vi "RandomFlag vs UUID Flag.vi"() -> ()   [LabVIEW 2020]
uses:
  <userlib>/_NEVSTOP/Communicable State Machine(CSM)/Communicable State Machine.lvlib
panel:
  out "UUID Flag":string
  out "Random Flag":u64
  out "unit (ms) 2":dbl[](graph)
  out "inside 2":i32
  out "outside 2":i32
  out "inside":i32
  out "outside":i32
  out "unit (ms)":dbl[][](graph)
  # "RandomFlag vs UUID Flag.vi"
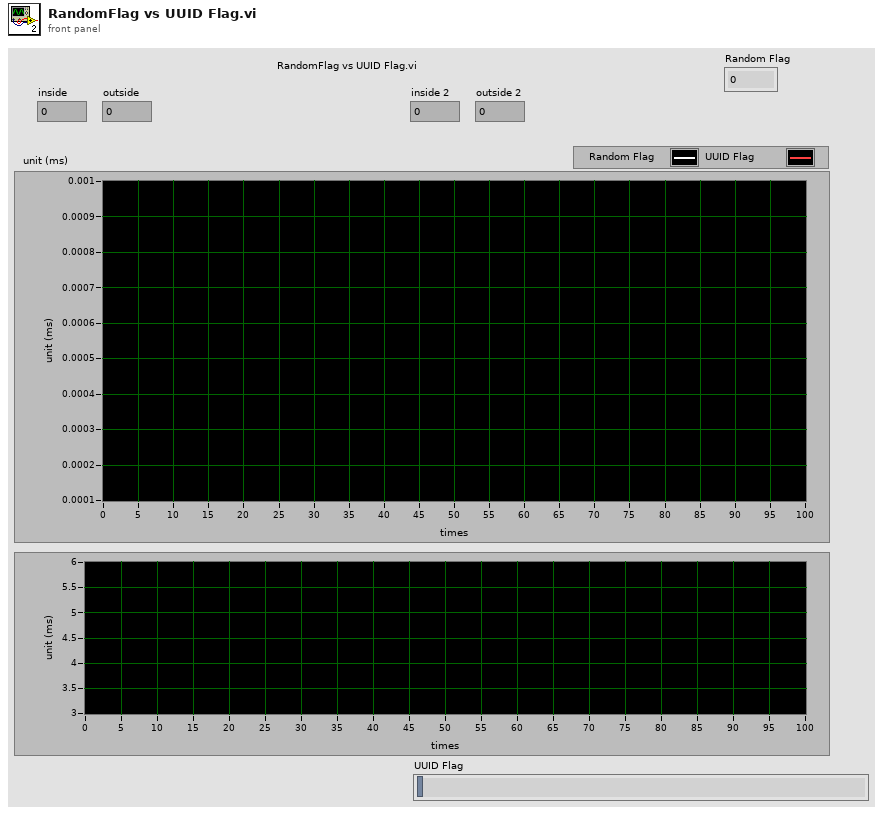
[diagram p1: front panel]
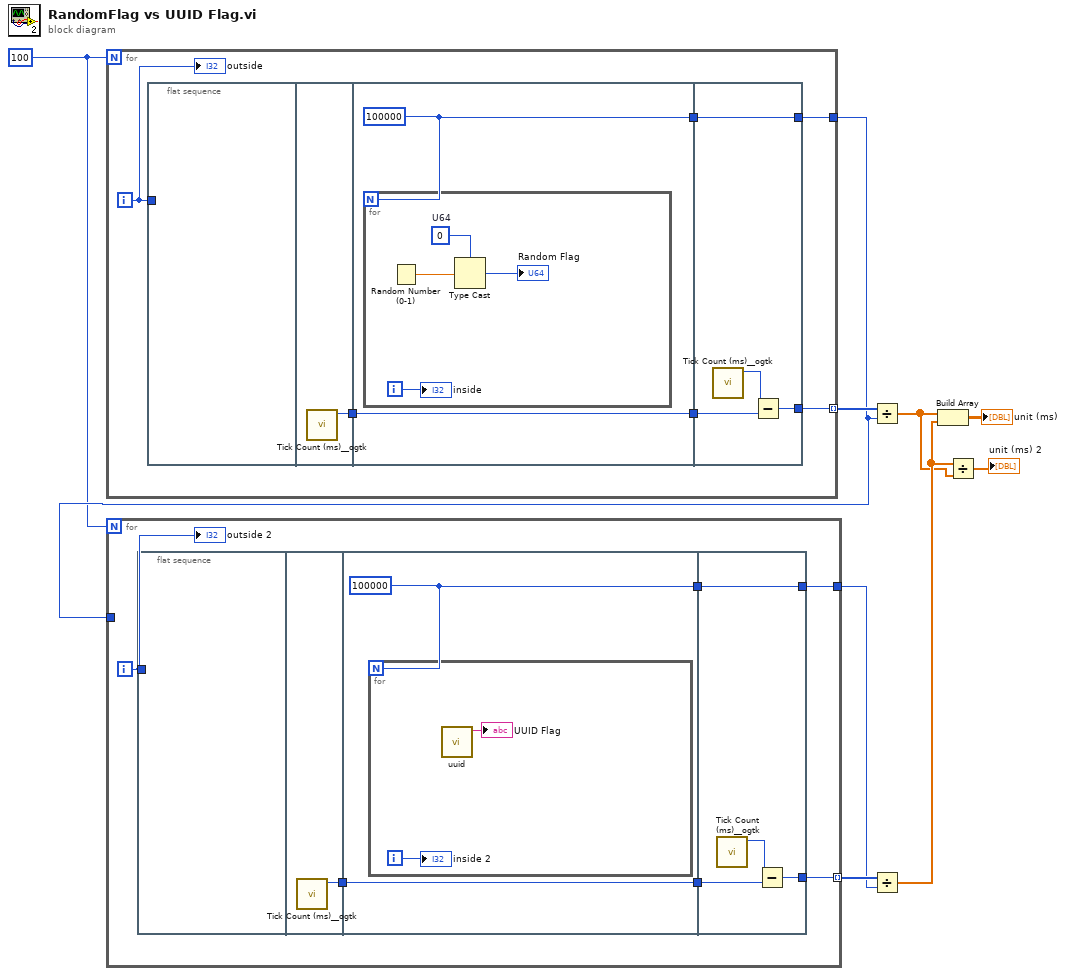
[diagram p0: block diagram]
diagram:
  w4 = 100
  n1 = for {
    N: w4 -> [_]
    tunnel: [w13] -> w9 mode=indexing
    tunnel: [w12] -> w5
    i -> [w10]
    n2 = flat-sequence {
      tunnel: w10 -> [_]
      tunnel: [w16] -> w15
      tunnel: w15 -> [w18]
      tunnel: [w18] -> w14
      tunnel: [w17] -> w11
      tunnel: w14 -> [w25]
      tunnel: [w24] -> w13
      tunnel: [w23] -> w12
      tunnel: w11 -> [w23]
      frame #0 {
      }
      frame #1 {
        n3 = call <userlib>:"Tick Count (ms)__ogtk.vi"() -> ("millisecond timer value"=w16:u32)  [unwired: 10 in, 1 out]
      }
      frame #2 {
        w17 = 100000
        n4 = for {
          N: w17 -> [_]
          i -> [w22]
          w19 = u64 0  # U64
          n5 = Random Number (0-1)() -> (number: 0 to 1=w21:dbl)
          n6 = Type Cast(type=w19, x=w21) -> (*(type *) &x=→"Random Flag":u64)
          "inside" <- w22
        }
      }
      frame #3 {
        n7 = call <userlib>:"Tick Count (ms)__ogtk.vi"() -> ("millisecond timer value"=w26:u32)  [unwired: 10 in, 1 out]
        n8 = Subtract(x=w26, y=w25) -> (x-y=w24:u32)
      }
    }
    "outside" <- w10
  }
  n9 = for {
    N: w4 -> [_]
    tunnel: [w30] -> w7 mode=indexing
    tunnel: [w29] -> w6
    tunnel: w5 -> [_]
    i -> [w27]
    n10 = flat-sequence {
      tunnel: w27 -> [_]
      tunnel: [w33] -> w32
      tunnel: w32 -> [w35]
      tunnel: [w35] -> w31
      tunnel: [w34] -> w28
      tunnel: w31 -> [w40]
      tunnel: [w39] -> w30
      tunnel: [w38] -> w29
      tunnel: w28 -> [w38]
      frame #0 {
      }
      frame #1 {
        n11 = call <userlib>:"Tick Count (ms)__ogtk.vi"() -> ("millisecond timer value"=w33:u32)  [unwired: 10 in, 1 out]
      }
      frame #2 {
        w34 = 100000
        n12 = for {
          N: w34 -> [_]
          i -> [w37]
          n13 = call <userlib>:"uuid.vi"() -> ("UUID"=→"UUID Flag":string)  [unwired: 11 in]
          "inside 2" <- w37
        }
      }
      frame #3 {
        n14 = call <userlib>:"Tick Count (ms)__ogtk.vi"() -> ("millisecond timer value"=w41:u32)  [unwired: 10 in, 1 out]
        n15 = Subtract(x=w41, y=w40) -> (x-y=w39:u32)
      }
    }
    "outside 2" <- w27
  }
  n16 = Divide(x=w9, y=w5) -> (x/y=w2:dbl[])
  n17 = Divide(x=w7, y=w6) -> (x/y=w3:dbl[])
  n18 = Build Array(w2, w3) -> (→"unit (ms)":dbl[][])
  n19 = Divide(x=w3, y=w2) -> (x/y=→"unit (ms) 2":dbl[])
